vi "Error Case.vi"   [LabVIEW 2020]
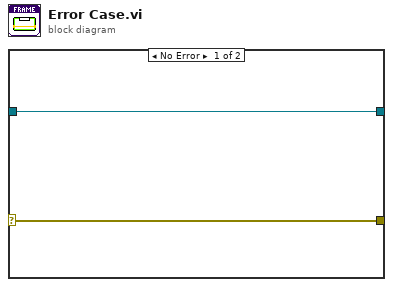
[diagram p0: block diagram]
diagram:
  n1 = case shown="No Error" {
    selector: _ -> [w2 w4]
    tunnel: [w2 w4] -> _
    tunnel: _ -> [w1 w3]
    tunnel: [w1 w3] -> _
    frame No Error {
    }
    frame Error {
    }
  }
